vi "IOL Master Disconnected 6003--error.vi"(11 "Master Key":string) -> (0 "error out":errorcluster)   [LabVIEW 2024, in "IOLink.lvlib"]
uses:
  IOLink.lvlib
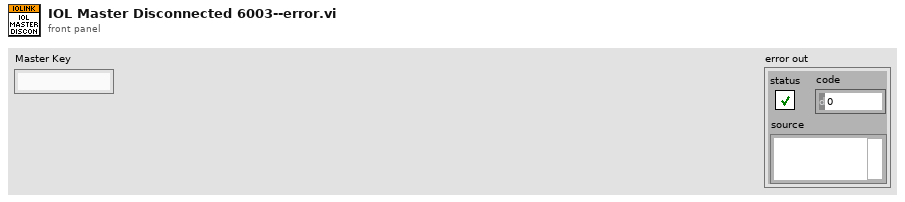
[diagram p1: front panel]
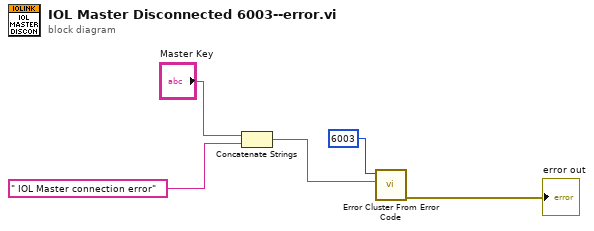
[diagram p0: block diagram]
diagram:
  n1 = Concatenate Strings("Master Key", " IOL Master connection error" ("string")) -> (w5:string)
  n2 = call <vilib>:"Error Cluster From Error Code.vi"("error message (\"\")"=w5, "error code (0)"=6003) -> ("error out"=→"error out":errorcluster)  [unwired: 7 in]
